vi "Read_Visa_Buffer.vi"(5 "Buffer In":string, 6 "error in (no error)":errorcluster, 8 "delay before read (ms)":u32=100, 9 "VISA Refnum in":refnum<visa-resource-name>) -> (0 "error out":errorcluster, 2 "Read":bool, 3 "VISA Refnum out":refnum<visa-resource-name>, 4 "Buffer Out":string)   [LabVIEW 2020]
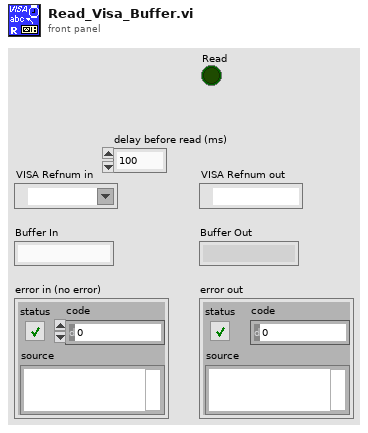
[diagram p1: front panel]
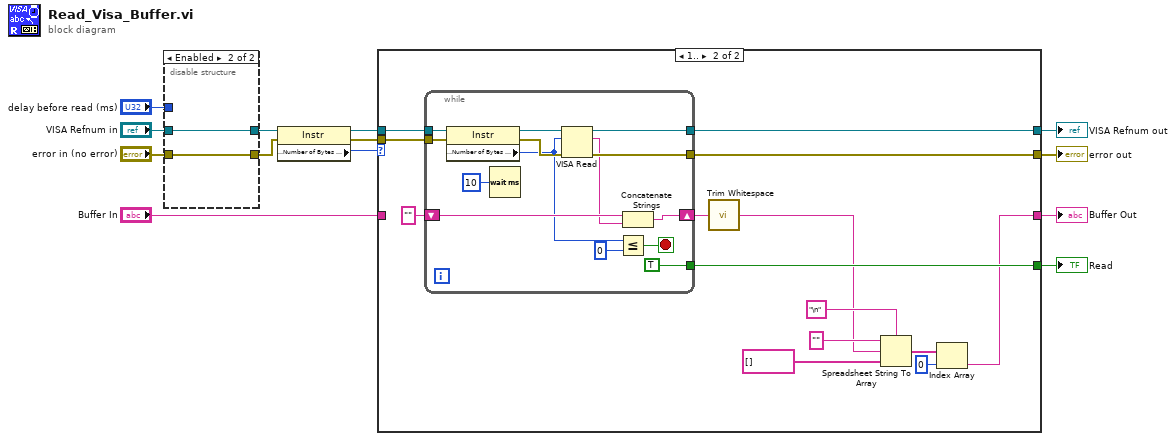
[diagram p0: block diagram]
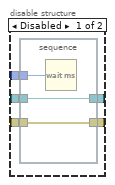
[diagram p2: hidden frame]
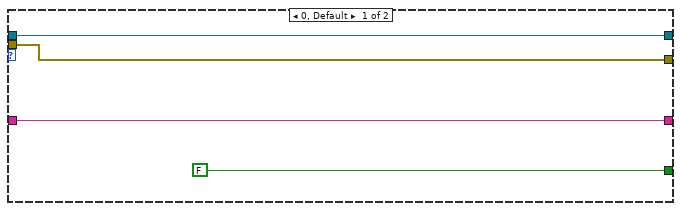
[diagram p3: hidden frame]
diagram:
  n1 = disable-structure shown="Enabled" {
    disable-tunnel: "VISA Refnum in" -> [w18 w23]
    disable-tunnel: [w17 w23] -> w5
    disable-tunnel: "error in (no error)" -> [w16 w22]
    disable-tunnel: [w15 w22] -> w3
    disable-tunnel: "delay before read (ms)" -> [w14 _]
    frame Disabled {
      n2 = stacked-sequence {
        tunnel: w18 -> [w21]
        tunnel: [w21] -> w17
        tunnel: w16 -> [w20]
        tunnel: [w20] -> w15
        tunnel: w14 -> [w19]
        frame #0 {
          n3 = Wait (ms)(milliseconds to wait=w19) -> ()  [unwired: 1 out]
        }
      }
    }
    frame Enabled {
    }
  }
  n4 = property class="Instr"(reference=w5, error in=w3) -> (reference out=w11:refnum<visa-resource-name>, error out=w12:errorcluster, "Serial Settings:Number of Bytes at Serial Port"=w13:u32)
  n5 = case shown="1.." w13 {
    tunnel: [w26 w41] -> w7
    tunnel: [w27 w28] -> w8
    tunnel: w11 -> [w27 w40]
    tunnel: w12 -> [w26 w39]
    tunnel: [w25 w29] -> w9
    tunnel: "Buffer In" -> [w25 _]
    tunnel: [FALSE ("x <= y?") w36] -> w1
    frame 0, Default {
    }
    frame 1.. {
      n6 = while {
        tunnel: [w55] -> w41
        tunnel: [w54] -> w28
        tunnel: w40 -> [w53]
        tunnel: w39 -> [w51]
        shift-right: [w46] -> w37
        shift-left: "" ("read buffer") -> [w48]
        tunnel: [TRUE ("x <= y?")] -> w36
        stop <- w49 stop-if-true
        n7 = property class="Instr"(reference=w53, error in=w51) -> (reference out=w52:refnum<visa-resource-name>, error out=w50:errorcluster, "Serial Settings:Number of Bytes at Serial Port"=w44:u32)
        n8 = Wait (ms)(milliseconds to wait=u32 10) -> ()  [unwired: 1 out]
        n9 = VISA Read(VISA resource name=w52, byte count=w44, error in (no error)=w50) -> (VISA resource name out=w54:refnum<visa-resource-name>, read buffer=w47:string, error out=w55:errorcluster)  [unwired: 1 out]
        n10 = Less Or Equal?(x=w44, y=u32 0) -> (x <= y?=w49:bool)
        n11 = Concatenate Strings(w48, w47) -> (w46:string)
      }
      n12 = call <vilib>:"Trim Whitespace.vi"("string"=w37) -> ("trimmed string"=w30:string)  [unwired: 1 in]
      n13 = Spreadsheet String To Array(delimiter (Tab)="\n", format string="", spreadsheet string=w30, array type (2D Dbl)=string[] []) -> (array=w32:string[])
      n14 = Index Array(array=w32, index=0) -> (element=w29:string)
    }
  }
  "Buffer Out" <- w9
  "VISA Refnum out" <- w8
  "error out" <- w7
  "Read" <- w1
